vi "NDHX Flow Characteristics.vi"(0 "Cp of Air (J/kgK)":dbl, 1 "Air Average Viscosity (Pa-s)":dbl, 2 "Thermal Conductivity (W/m-K)":dbl, 3 "FLiNaK Viscosity (Pa-s)":dbl, 5 "Stack Inner Diameter":dbl, 7 "Air Mass Flow (kg/s)":dbl, 9 "Pipe Diameter (m)":dbl, 12 "Cp of FLiNaK (J/kgK)":dbl, 13 "Thermal Conductivity of FLiNaK (W/m-K)":dbl, 14 "Sec Mass Flow (kg/s)":dbl) -> (4 "Air Re":dbl, 6 "Sec Re":dbl, 8 "Air Pr":dbl, 10 "Sec Pr":dbl, 15 "Air Mass Flux (kg/s-m^2)":dbl)   [LabVIEW 2019]
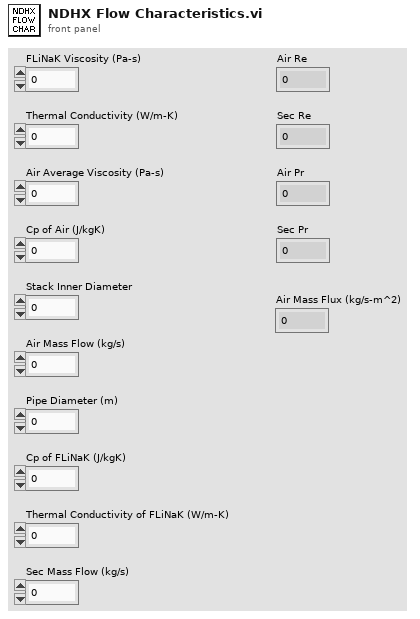
[diagram p1: front panel]
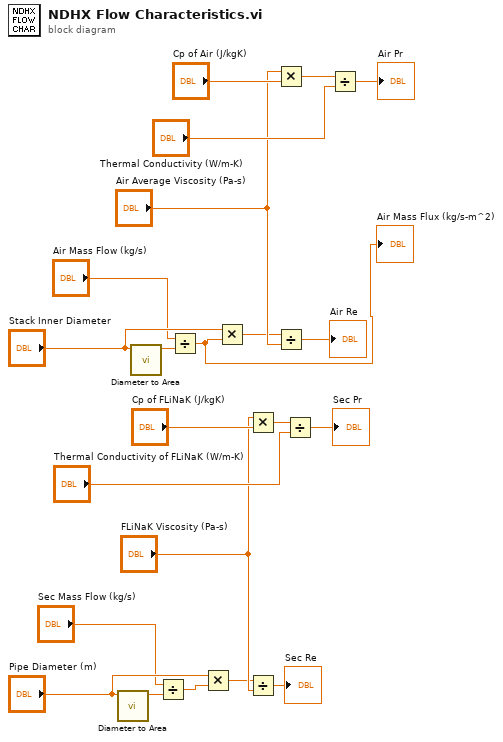
[diagram p0: block diagram]
diagram:
  n1 = call "Diameter to Area.vi"("Diameter (m)"="Pipe Diameter (m)") -> ("Area (m^2)"=w3:dbl)  [unwired: 10 in]
  n2 = call "Diameter to Area.vi"("Diameter (m)"="Stack Inner Diameter") -> ("Area (m^2)"=w5:dbl)  [unwired: 10 in]
  n3 = Divide(x="Sec Mass Flow (kg/s)", y=w3) -> (x/y=w6:dbl)
  n4 = Divide(x="Air Mass Flow (kg/s)", y=w5) -> (x/y=w1:dbl)
  "Air Mass Flux (kg/s-m^2)" <- w1
  n5 = Multiply(x="Pipe Diameter (m)", y=w6) -> (x*y=w10:dbl)
  n6 = Multiply(x="Stack Inner Diameter", y=w1) -> (x*y=w9:dbl)
  n7 = Multiply(x="FLiNaK Viscosity (Pa-s)", y="Cp of FLiNaK (J/kgK)") -> (x*y=w16:dbl)
  n8 = Divide(x=w10, y="FLiNaK Viscosity (Pa-s)") -> (x/y=→"Sec Re":dbl)
  n9 = Multiply(x="Air Average Viscosity (Pa-s)", y="Cp of Air (J/kgK)") -> (x*y=w15:dbl)
  n10 = Divide(x=w9, y="Air Average Viscosity (Pa-s)") -> (x/y=→"Air Re":dbl)
  n11 = Divide(x=w16, y="Thermal Conductivity of FLiNaK (W/m-K)") -> (x/y=→"Sec Pr":dbl)
  n12 = Divide(x=w15, y="Thermal Conductivity (W/m-K)") -> (x/y=→"Air Pr":dbl)
